vi "WriteDataCluster.vi"(8 "error in (no error)":errorcluster, 10 "DataCluster":cluster{"CounterNum":i32}) -> (0 "error out":errorcluster)   [LabVIEW 2013, in "Data.lvclass"]
uses:
  Data.lvclass
  Data.lvclass/Data.ctl
  Singleton.lvclass/Singleton.lvclass/Singleton.ctl
  Singleton.lvclass/Constructor.vi
  Singleton.lvclass/Singleton.lvclass
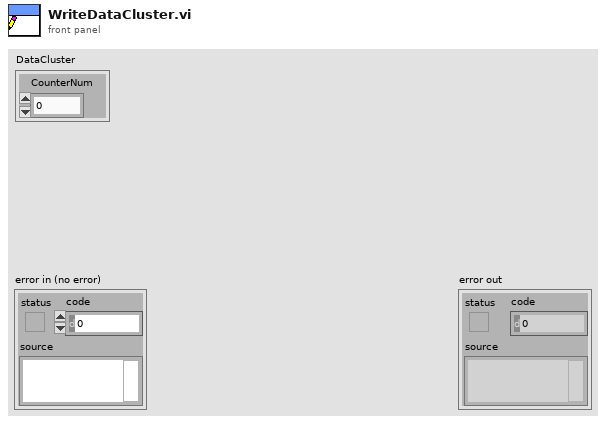
[diagram p1: front panel]
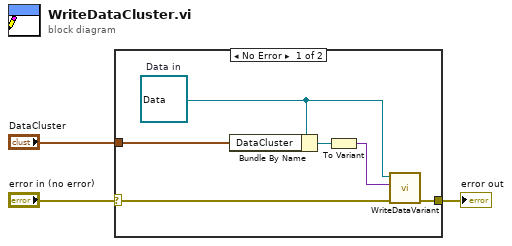
[diagram p0: block diagram]
diagram:
  n1 = case shown="No Error" "error in (no error)" {
    selector: "error in (no error)" -> [w4 w10]
    tunnel: [w7 w10] -> w2
    tunnel: "DataCluster" -> [w9 _]
    frame No Error {
      w5 = refnum<class "Data.lvclass"> refnum  # Data in
      n2 = Bundle By Name(cluster=w5, "DataCluster"=w9) -> (w8:refnum<class "Data.lvclass">)
      n3 = To Variant(anything=w8) -> (Variant=w6:variant)
      n4 = call "WriteDataVariant.vi"("error in (no error)"=w4, "DataVariant"=w6, "Singleton.lvclass In"=w5) -> ("error out"=w7:errorcluster)  [unwired: 7 in, 1 out]
    }
    frame Error {
    }
  }
  "error out" <- w2
